vi "Write Config.vi"(8 "error in (no error)":errorcluster, 9 "Re-Init?":bool, 10 "ICM File In":path, 11 "Polynomial in":refnum<class "Polynomial.lvclass">) -> (0 "error out":errorcluster, 3 "Polynomial out":refnum<class "Polynomial.lvclass">)   [LabVIEW 2015, in "Polynomial.lvclass"]
doc: "Polynomial.lvclass:Write Config.vi\n\nThis VI writes the Polynomial Class parameters to the ICM configuration file.\n\nInstrument Communication Module Version 1.0\nSeptember, 2017 Original Code Consulting David Thomson\n www.originalcode.com"
uses:
  Polynomial.lvclass
  Polynomial.lvclass/Polynomial.ctl
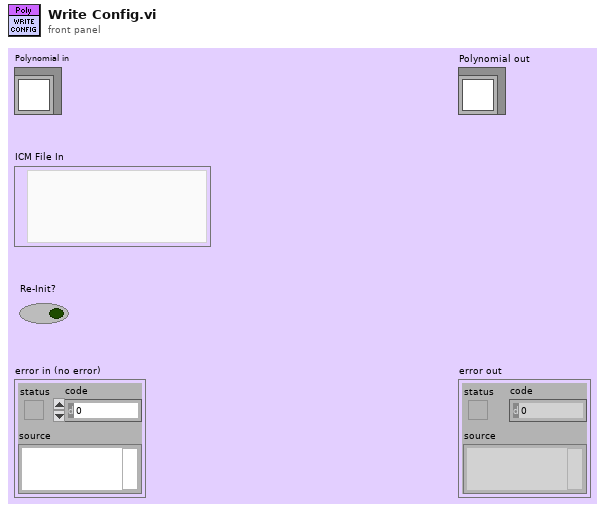
[diagram p1: front panel]
types:
  T1 = typedef "Polynomial Config.ctl" = cluster{"Polynomials":cluster{"Instance":string, "Polynomial":dbl[]}[]}
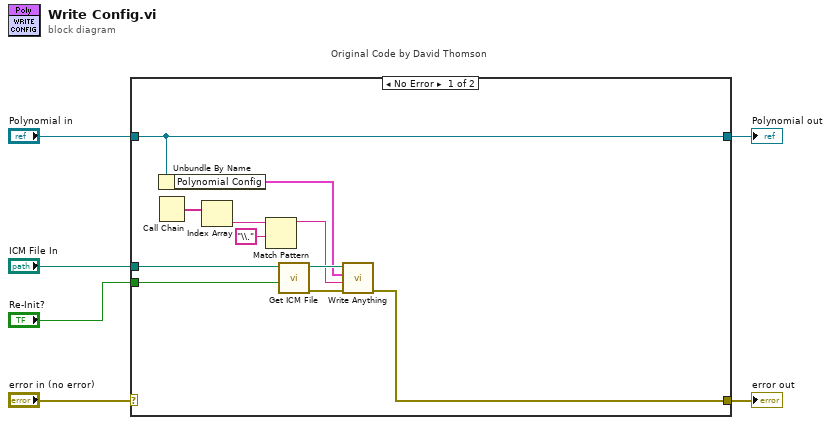
[diagram p0: block diagram]
diagram:
  n1 = case "Original Code by David Thomson" shown="No Error" "error in (no error)" {
    selector: "error in (no error)" -> [_ w19]
    tunnel: [w13 w19] -> w5
    tunnel: [w17 w18] -> w3
    tunnel: "Polynomial in" -> [w17 w18]
    tunnel: "ICM File In" -> [w12 _]
    tunnel: "Re-Init?" -> [w11 _]
    frame No Error {
      n2 = Call Chain() -> (call chain=w9:string[])
      n3 = Unbundle By Name(w17) -> ("Polynomial Config"=w14:T1)
      n4 = Index Array(array=w9) -> (element=w8:string)  [unwired: 1 in]
      n5 = Match Pattern(string=w8, regular expression="\\.") -> (before substring=w7:string)  [unwired: 1 in, 3 out]
      n6 = call "Get ICM File.vi"("Re-Init?"=w11, "ICM File In"=w12) -> ("error out"=w16:errorcluster, "ICM File"=w15:path)  [unwired: 8 in]
      n7 = call "Write Anything.vi"("Error In"=w16, "Section Name (Name of \"Anything\")"=w7, "Anything"=w14, "Path (dialog)"=w15) -> ("Error Out"=w13:errorcluster)  [unwired: 7 in]
    }
    frame Error {
    }
  }
  "error out" <- w5
  "Polynomial out" <- w3
